vi "SOAE Main Panel.vi"(0 "Expt State (in)":T1) -> (4 "Expt State out":T1)   [LabVIEW 2020]
uses:
  Utility VIs/Type Defs/Left-Right ring.ctl
  CFTS Main Panel SubVIs/CFTS-Experiment State.ctl
  <vilib>/printing/EasyPrintingControls.llb/layout_options.ctl
  <vilib>/printing/EasyPrintingControls.llb/orientation.ctl
  <vilib>/printing/EasyPrintingControls.llb/panel_scaling_for_page.ctl
  <vilib>/printing/EasyPrintingControls.llb/margins.ctl
  <vilib>/printing/EasyPrintingControls.llb/margin_values.ctl
  <vilib>/printing/EasyPrintingControls.llb/measurement_system.ctl
  <vilib>/printing/EasyPrintingControls.llb/printer_options.ctl
  <vilib>/printing/EasyPrintingControls.llb/printing_method.ctl
  <vilib>/printing/EasyPrintingControls.llb/color_or_monochrome.ctl
  <vilib>/printing/EasyPrintingControls.llb/page_header_options.ctl
  <vilib>/printing/EasyPrintingControls.llb/page_headers.ctl
  <vilib>/printing/EasyPrintingControls.llb/page_header_content_options.ctl
  Utility VIs/Buttons/KCheckmarkBoolean 2.ctl
  Typedefs/SOAE-Options.ctl
  Typedefs/SOAE-Parameters.ctl
  Typedefs/SOAE-State.ctl
  <vilib>/printing/EasyPrintingControls.llb/contents.ctl
  <vilib>/printing/EasyPrinting.llb/Easy Print VI Panel or Documentation (refnum).vi
  <vilib>/Utility/NIReport.llb/NI_ReportGenerationCore.lvlib
panel:
  out "Acquired":i32
  in  "Save raw data":T2
  in  "layout options":T3={"orientation (unchanged)"=0, "panel scaling for page (unchanged)"=0, "margins"={"override VI margins (false)"=FALSE, "margins (1.00)"={"top"=1.0, "left"=1.0, "right"=1.0, "bottom"=1.0}, "measurement system (default)"=0}, "printer options"={"destination printer name (current)"="", "printing method (unchanged)"=0, "color or monochrome (unchanged)"=0}, "page header options"={"page headers (unchanged)"=0, "page header content options"={"Include VI Name"=TRUE, "Include VI Path"=TRUE, "Include Last Modification Date"=TRUE, "Include Date Printed"=TRUE, "Include Page Number"=TRUE, "Include VI Icon"=TRUE}}} {"page header options"."page headers (unchanged)" items=["Unchanged", "Include page headers", "Do not include page headers"]; "printer options"."color or monochrome (unchanged)" items=["Unchanged", "Color/grayscale", "Monochrome"]; "printer options"."printing method (unchanged)" items=["Unchanged", "Standard", "PostScript", "Bitmap"]; "panel scaling for page (unchanged)" items=["Unchanged", "No Scaling", "Scale front panel to fit"]; "orientation (unchanged)" items=["Unchanged", "portrait", "landscape"]; "margins"."measurement system (default)" items=["Default", "US", "Metric"]; "margins"."margins (1.00)"."right" format="%.2f"; "margins"."margins (1.00)"."bottom" format="%.2f"; "margins"."margins (1.00)"."top" format="%.2f"; "margins"."margins (1.00)"."left" format="%.2f"}
  in  "Params":T16={"Ear"=enum."Right", "Sampling rate (Hz)"=0.25, "Number of FFT points"=37, "Number of averages"=5.0, "Smoothing binwidth (Hz)"=300.0, "Mic gain (dB)"=5.0}
  in  "Start":bool
  in  "Stop":bool
  out "User":string
  out "Run #":string
  out "ID #":u16
  out "finished":errorcluster
  in  "Listbox":i32(listbox)
  out "Spectrum":cluster{"X":dbl[], "X":dbl[]}[](graph)
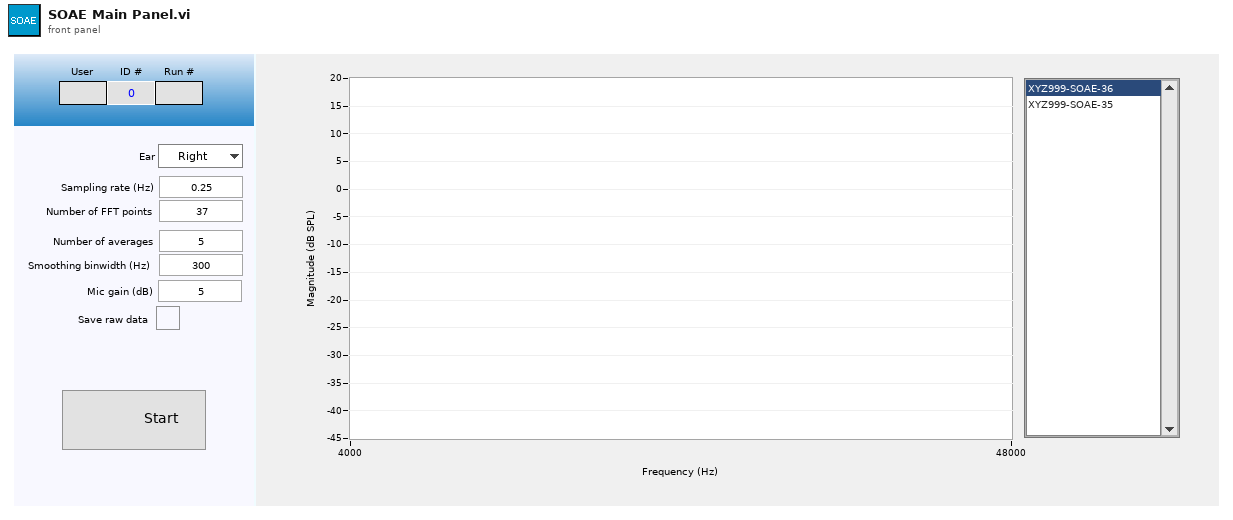
[diagram p1: front panel]
types:
  T1 = typedef "CFTS-Experiment State.ctl" = cluster{"Experimenter":string, "Number":u32, "Right":string, "Left":string, "Data Folder":path, "State File":path, "Version Info":string, "End Exposure Time":dbl, "Exposure Duration":string, "Run #":cluster{"CAP":i16, "ABR":i16, "DP":i16, "VsEP":i16, "MeasSeq":i16, "SubSeq":i16, "SFOAE":i16}}
  T2 = typedef "KCheckmarkBoolean 2.ctl" = bool
  T3 = typedef "NI_ReportGenerationCore.lvlib/layout_options.ctl" = cluster{"orientation (unchanged)":T4, "panel scaling for page (unchanged)":T5, "margins":T6, "printer options":T9, "page header options":T12}
  T4 = typedef "NI_ReportGenerationCore.lvlib/orientation.ctl" = u16
  T5 = typedef "NI_ReportGenerationCore.lvlib/panel_scaling_for_page.ctl" = u16
  T6 = typedef "NI_ReportGenerationCore.lvlib/margins.ctl" = cluster{"override VI margins (false)":bool, "margins (1.00)":T7, "measurement system (default)":T8}
  T7 = typedef "NI_ReportGenerationCore.lvlib/margin_values.ctl" = cluster{"top":dbl, "left":dbl, "right":dbl, "bottom":dbl}
  T8 = typedef "NI_ReportGenerationCore.lvlib/measurement_system.ctl" = u16
  T9 = typedef "NI_ReportGenerationCore.lvlib/printer_options.ctl" = cluster{"destination printer name (current)":string, "printing method (unchanged)":T10, "color or monochrome (unchanged)":T11}
  T10 = typedef "NI_ReportGenerationCore.lvlib/printing_method.ctl" = u16
  T11 = typedef "NI_ReportGenerationCore.lvlib/color_or_monochrome.ctl" = u16
  T12 = typedef "NI_ReportGenerationCore.lvlib/page_header_options.ctl" = cluster{"page headers (unchanged)":T13, "page header content options":T14}
  T13 = typedef "NI_ReportGenerationCore.lvlib/page_headers.ctl" = u16
  T14 = typedef "NI_ReportGenerationCore.lvlib/page_header_content_options.ctl" = cluster{"Include VI Name":bool, "Include VI Path":bool, "Include Last Modification Date":bool, "Include Date Printed":bool, "Include Page Number":bool, "Include VI Icon":bool}
  T15 = typedef "Left-Right ring.ctl" = enum16{"Right", "Left"}
  T16 = cluster{"Ear":T15, "Sampling rate (Hz)":dbl, "Number of FFT points":i32, "Number of averages":dbl, "Smoothing binwidth (Hz)":dbl, "Mic gain (dB)":dbl}
  T17 = typedef "SOAE-State.ctl" = cluster{"aborted":bool, "files":path[]}
  T18 = typedef "SOAE-Parameters.ctl" = cluster{"Ear":enum16{"Right", "Left"}, "Fs (Hz)":dbl, "Nfft":i32, "Navg":i32, "Binwidth (Hz)":dbl, "Gain (dB)":dbl}
  T19 = typedef "SOAE-Options.ctl" = cluster{"FreqScale":cluster{"Min":dbl, "Max":dbl}, "save raw":bool}
  T20 = typedef "SOAE-Acq Runtime.ctl" = cluster{"freq":dbl[], "raw":dbl[], "mag":dbl[], "pt":dbl[], "path":path, "task":refnum<k21>, "nacq":i32, "gain":dbl, "navg":i32, "stream":refnum<file>, "nread":i32, "fir":dbl[]}
  T21 = enum8{"Enabled", "Disabled", "Disabled and Grayed Out"}
  T22 = typedef "NI_ReportGenerationCore.lvlib/contents.ctl" = u16
  T23 = cluster{"Ear":T15, "Fs (Hz)":dbl, "Nfft":i32, "Number of averages":dbl, "Binwidth (Hz)":dbl, "Gain (dB)":dbl}
  T24 = cluster{"Params":cluster{"Ear":T15, "Fs (Hz)":dbl, "Nfft":i32, "Number of averages":dbl, "Binwidth (Hz)":dbl, "Gain (dB)":dbl}, "Path out":path, "save raw":bool}
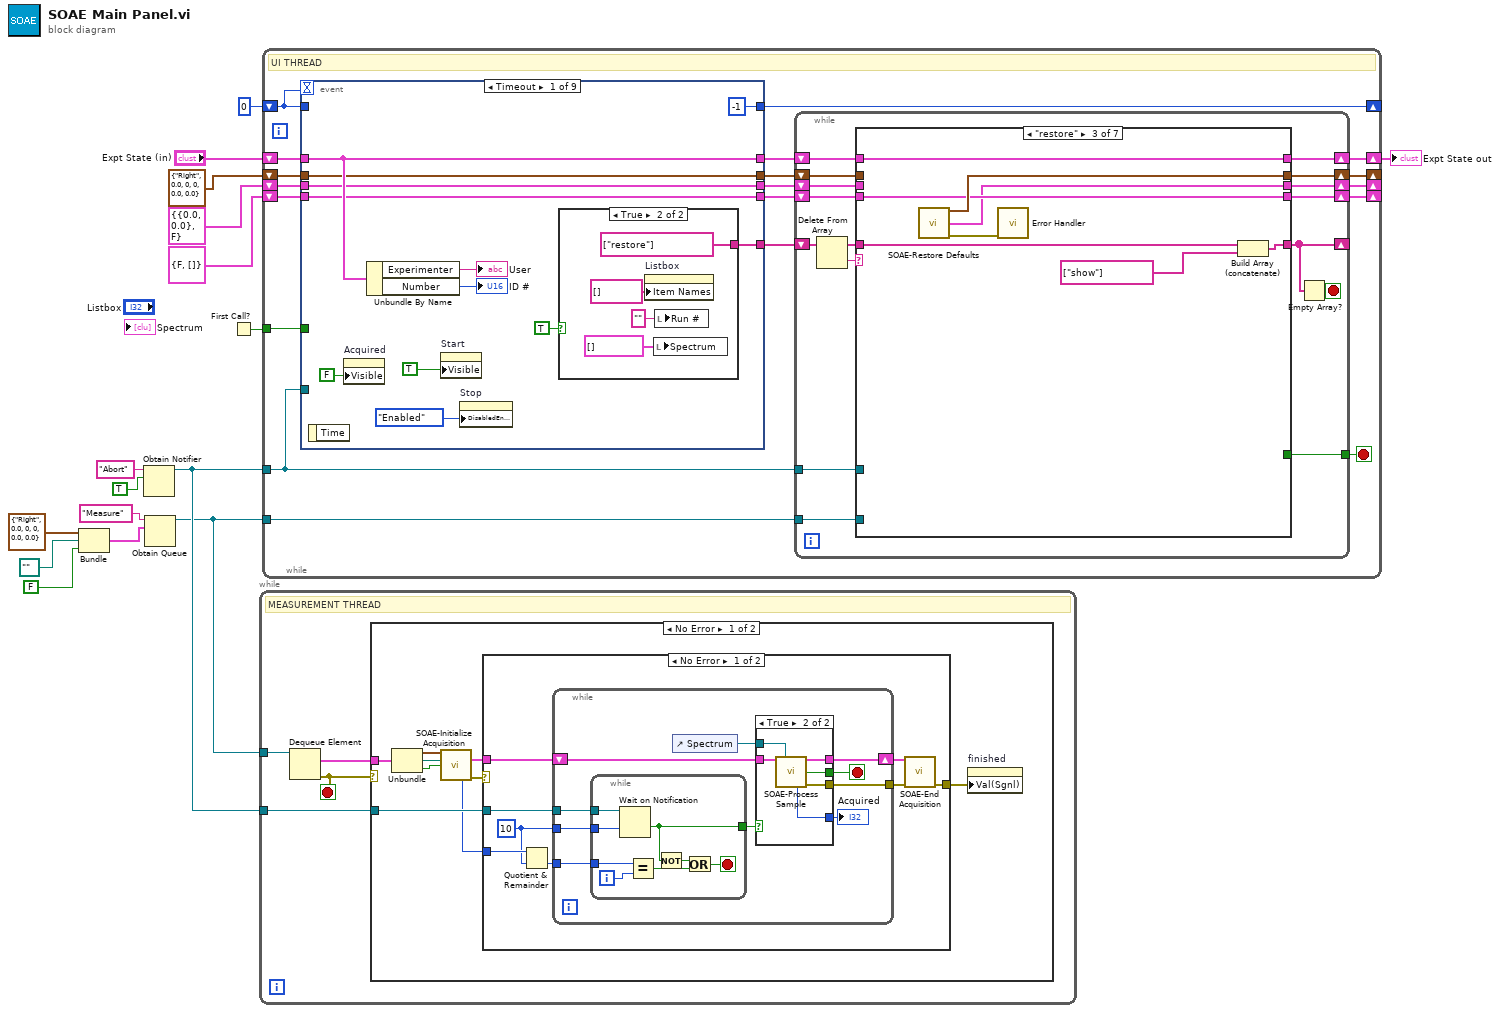
[diagram p0: block diagram]
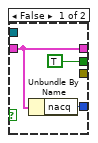
[diagram p2: hidden frame]
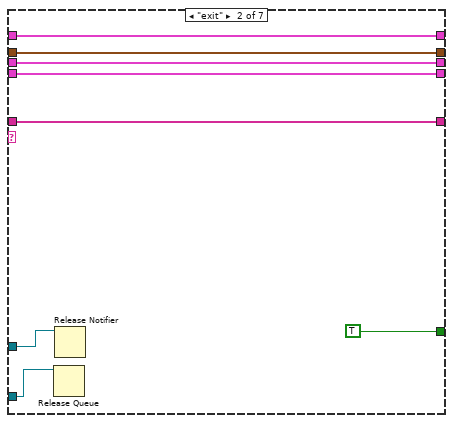
[diagram p6: hidden frame]
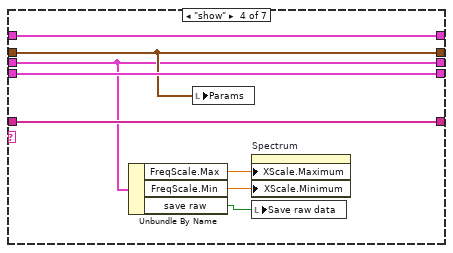
[diagram p7: hidden frame]
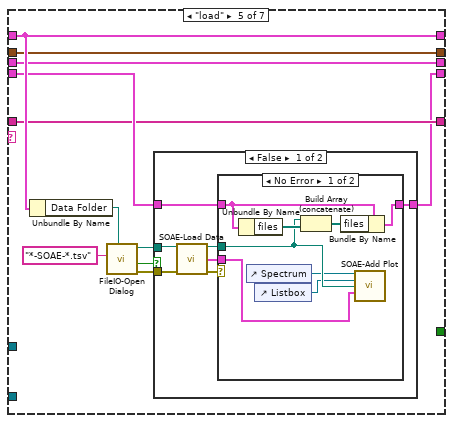
[diagram p8: hidden frame]
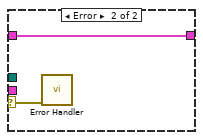
[diagram p9: hidden frame]
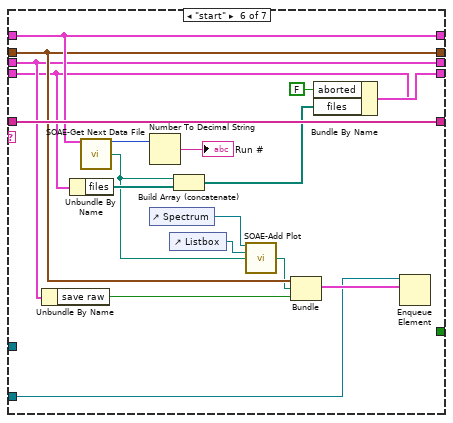
[diagram p11: hidden frame]
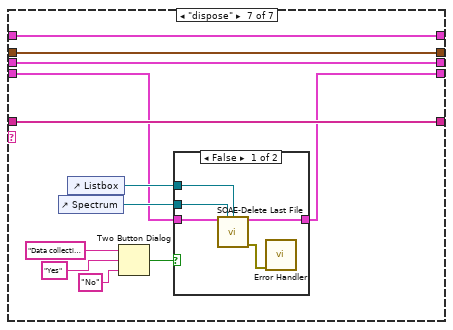
[diagram p12: hidden frame]
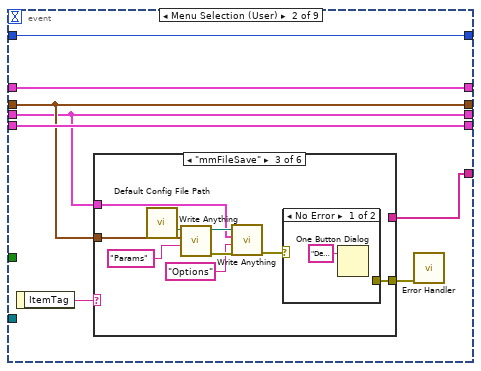
[diagram p15: hidden frame]
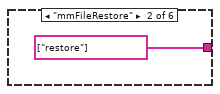
[diagram p17: hidden frame]
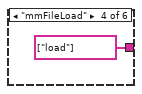
[diagram p19: hidden frame]
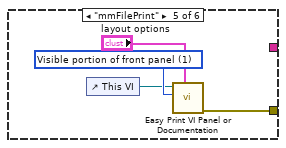
[diagram p20: hidden frame]
diagram:
  n1 = Bundle("Params"=T18 {"Ear"=enum."Right", "Fs (Hz)"=0.0, "Nfft"=0, "Navg"=0, "Binwidth (Hz)"=0.0, "Gain (dB)"=0.0}, path "", FALSE) -> (w12:cluster{"Params":T18, path, bool})  [unwired: 1 in]
  n2 = Obtain Notifier(name (unnamed)="Abort", notification data type=TRUE) -> (notifier out=w15:refnum<notifier>)  [unwired: 2 in, 2 out]
  n3 = Obtain Queue(name (unnamed)="Measure", element data type=w12) -> (queue out=w8:refnum<queue>)  [unwired: 3 in, 2 out]
  n4 = First Call?() -> (First Call?: T/F=w11:bool)
  n5 = while {
    tunnel: w8 -> [w20]
    tunnel: w15 -> [w17]
    stop <- w19 stop-if-true
    # "MEASUREMENT THREAD"
    n6 = Dequeue Element(queue=w20) -> (element=w18:cluster{"Params":T18, path, bool}, error out=w19:errorcluster)  [unwired: 2 in, 2 out]
    n7 = case shown="No Error" w19 {
      tunnel: w18 -> [w29 _]
      tunnel: w17 -> [w28 _]
      frame No Error {
        n8 = Unbundle(w29) -> ("Params"=w25:T18, w24:path, w27:bool)
        n9 = call "SOAE-Initialize Acquisition.vi"("Params"=w25, "Path"=w24, "raw data"=w27) -> ("runtime"=w23:T20, "T (ms)"=w22:u32, "error out"=w26:errorcluster)  [unwired: 10 in]
        n10 = case shown="No Error" w26 {
          selector: w26 -> [_ w65]
          tunnel: w28 -> [w37 _]
          tunnel: w23 -> [w36 _]
          tunnel: w22 -> [w35 _]
          tunnel: [w30 w65] -> w21
          frame No Error {
            w34 = 10 ("timeout in ms (-1)")
            n11 = Quotient & Remainder(x=w35, y=w34) -> (floor(x/y)=w33:u32)  [unwired: 1 out]
            n12 = while {
              shift-right: [w43] -> w31
              shift-left: w36 -> [w44]
              tunnel: w37 -> [w47]
              tunnel: w34 -> [w46]
              tunnel: w33 -> [w45]
              tunnel: [w40] -> w32
              stop <- w41 stop-if-true
              n13 = while {
                tunnel: [w58] -> w42
                tunnel: w46 -> [w63]
                tunnel: w45 -> [w62]
                tunnel: w47 -> [w64]
                i -> [w61]
                stop <- w59 stop-if-true
                n14 = Wait on Notification(notifier=w64, timeout in ms (-1)=w63) -> (timed out?=w58:bool)  [unwired: 2 in, 3 out]
                n15 = Equal?(x=w62, y=w61) -> (x = y?=w60:bool)
                n16 = Not(x=w58) -> (.not. x?=w57:bool)
                n17 = Or(x=w57, y=w60) -> (x .or. y?=w59:bool)
              }
              n18 = control-ref of="Spectrum"() -> (w39:refnum<vi>)
              n19 = case shown="True" w42 {
                tunnel: w44 -> [w49 w56]
                tunnel: [w49 w55] -> w43
                tunnel: [TRUE w53] -> w41
                tunnel: [_ w54] -> w40
                tunnel: w39 -> [_ w52]
                tunnel: [w48 w51] -> w38
                frame False {
                  n20 = Unbundle By Name(w49) -> ("nacq"=w48:i32)
                }
                frame True {
                  n21 = call "SOAE-Process Sample.vi"("runtime in"=w56, "Graph"=w52) -> ("runtime out"=w55:T20, "finished"=w53:bool, "acquired"=w51:i32, "error out"=w54:errorcluster)  [unwired: 10 in]
                }
              }
              "Acquired" <- w38
            }
            n22 = call "SOAE-End Acquisition.vi"("runtime"=w31, "error in (no error)"=w32) -> ("error out"=w30:errorcluster)  [unwired: 13 in]
          }
          frame Error {
          }
        }
        n23 = property on="finished" class="Clust (strict)"("Val(Sgnl)"=w21) -> ()  [unwired: 2 in, 2 out]
      }
      frame Error {
      }
    }
  }
  n24 = while {
    tunnel: w8 -> [w69]
    shift-right: [w84] -> _
    shift-left: 0 -> [w80]
    tunnel: w11 -> [w83]
    shift-right: [w75] -> w2
    shift-left: "Expt State (in)" -> [w82]
    shift-right: [w77] -> _
    shift-left: T18 {"Ear"=enum."Right", "Fs (Hz)"=0.0, "Nfft"=0, "Navg"=0, "Binwidth (Hz)"=0.0, "Gain (dB)"=0.0} ("Params") -> [w81]
    shift-right: [w71] -> _
    shift-left: T17 {"aborted"=FALSE, "files"=[]} ("State") -> [w73]
    tunnel: w15 -> [w70]
    shift-right: [w66] -> _
    shift-left: T19 {"FreqScale"={"Min"=0.0, "Max"=0.0}, "save raw"=FALSE} ("Options") -> [w68]
    stop <- w74 stop-if-true
    # "UI THREAD"
    n25 = event shown="[0] Timeout" {
      selector: _ -> [_ _ _ _ _ _ _ _ _]
      dyn-events: _ -> [_ _ _ _ _ _ _ _ _]
      timeout: w80 -> [_ _ w243 _ _ _ _ _ _]
      tunnel: [-1 w216 w243 w248 w255 w263 w274 w288 w297] -> w84
      tunnel: w83 -> [_ _ _ _ _ _ _ _ _]
      tunnel: w82 -> [w205 w215 w239 w247 w254 w262 w273 w287 w296]
      tunnel: [w205 w215 w239 w247 w254 w262 w273 w287 w296] -> w76
      tunnel: w81 -> [w204 w212 w241 _ w253 w264 w275 w286 w295]
      tunnel: [w204 w212 w241 "Params" w253 w264 w275 w286 w295] -> w78
      tunnel: w80 -> [_ w216 _ w248 w255 w263 w274 w288 w297]
      tunnel: [w200 w214 string[] ["exit"] ("f") _ _ string[] ["start"] ("f") _ w277 _] -> w79
      tunnel: w73 -> [w203 w213 w238 w246 w252 w260 w272 w281 w294]
      tunnel: [w203 w213 w238 w246 w252 w260 w267 w281 w294] -> w72
      tunnel: w70 -> [_ _ _ _ _ w259 w271 _ _]
      tunnel: w68 -> [w197 w211 w237 w244 w251 w258 w268 w285 w293]
      tunnel: [w197 w211 w237 w244 w250 w258 w268 w285 w292] -> w67
      event Timeout {
        n26 = event-data() -> ()  [unwired: 1 in, 1 out]
        n27 = property on="Acquired" class="DigNum (strict)"("Visible"=FALSE) -> ()  [unwired: 2 in, 2 out]
        n28 = Unbundle By Name(w205) -> ("Experimenter"=→"User":string, "Number"=→"ID #":u32)
        n29 = property on="Start" class="Bool"("Visible"=TRUE) -> ()  [unwired: 2 in, 2 out]
        n30 = property on="Stop" class="Bool"("DisabledEnum"=T21."Enabled" ("Disabled")) -> ()  [unwired: 2 in, 2 out]
        n31 = case shown="True" TRUE {
          tunnel: [_ string[] ["restore"]] -> w200
          frame False {
          }
          frame True {
            n32 = property on="Listbox" class="LstBox (strict)"("Item Names"=string[] []) -> ()  [unwired: 2 in, 2 out]
            n33 = local write "Spectrum"(cluster{"X":dbl[], "X":dbl[]}[] [] ("Spectrum")) -> ()
            n34 = local write "Run #"("" ("Run #")) -> ()
          }
        }
      }
      event Menu Selection (User) {
        n35 = event-data() -> ("ItemTag"=w218:string)  [unwired: 1 in]
        n36 = case shown="\"mmFileSave\"" w218 {
          tunnel: [_ _ w225 _ w232 _] -> w217
          tunnel: w212 -> [_ _ w226 _ _ _]
          tunnel: [_ string[] ["restore"] _ string[] ["load"] _ string[] ["exit"]] -> w214
          tunnel: w211 -> [_ _ w221 _ _ _]
          frame "", Default {
          }
          frame "mmFileRestore" {
          }
          frame "mmFileSave" {
            n37 = call "Default Config File Path.vi"() -> ("Default config file name"=w228:path)
            n38 = call "Write Anything.vi"("Section Name (Name of \"Anything\")"="Params" ("Section Name (Name of \"Anything\")"), "Anything"=w226, "Path (dialog)"=w228) -> ("Error Out"=w224:errorcluster, "Path out"=w223:path)  [unwired: 7 in]
            n39 = call "Write Anything.vi"("Error In"=w224, "Section Name (Name of \"Anything\")"="Options" ("Section Name (Name of \"Anything\")"), "Anything"=w221, "Path (dialog)"=w223) -> ("Error Out"=w220:errorcluster)  [unwired: 6 in, 1 out]
            n40 = case shown="No Error" w220 {
              selector: w220 -> [_ w230]
              tunnel: [_ w230] -> w225
              frame No Error {
                n41 = One Button Dialog(message="Defaults saved.") -> ()  [unwired: 1 in, 1 out]
              }
              frame Error {
              }
            }
          }
          frame "mmFileLoad" {
          }
          frame "mmFilePrint" {
            w234 = T22 1 items=["Complete front panel", "Visible portion of front panel", "Icon, description, panel and diagram", "Documentation: Using the panel", "Documentation: Using as a subVI", "Documentation: Complete", "Documentation: Custom"] ("contents (complete front panel)")
            n42 = control-ref of="This VI"() -> (w233:refnum<vi>)
            n43 = call-poly <vilib>:"Easy Print VI Panel or Documentation.vi"("layout options"="layout options", "contents (complete front panel)"=w234, "VI reference"=w233) -> ("error out"=w232:errorcluster)  [unwired: 7 in, 1 out]
          }
          frame "mmFileExit" {
          }
        }
        n44 = call "Error Handler.vi"("error in (no error)"=w217) -> ()  [unwired: 13 in, 2 out]
      }
      event Panel Close? {
        n45 = event-data() -> ()  [unwired: 1 in, 1 out]
        n46 = event-data("Discard?"=TRUE) -> ()  [unwired: 1 in, 1 out]
      }
      event "Params": Value Change {
        n47 = event-data() -> ()  [unwired: 1 in, 1 out]
      }
      event Value Change {
        n48 = event-data() -> ()  [unwired: 1 in, 1 out]
        n49 = Bundle By Name(cluster=w251, "save raw"="Save raw data") -> (w250:T19)
      }
      event "Start": Value Change {
        n50 = event-data() -> ()  [unwired: 1 in, 1 out]
        n51 = Cancel Notification(0:w259) -> ()  [unwired: 1 in, 3 out]
        n52 = property on="Start" class="Bool"("Visible"=FALSE) -> ()  [unwired: 2 in, 2 out]
        n53 = property on="Acquired" class="DigNum (strict)"("Visible"=TRUE) -> ()  [unwired: 2 in, 2 out]
        n54 = local write "Acquired"(0 ("Acquired")) -> ()
      }
      event "Stop": Value Change {
        n55 = event-data() -> ()  [unwired: 1 in, 1 out]
        n56 = Send Notification(notification=TRUE, notifier=w271) -> ()  [unwired: 1 in, 2 out]
        n57 = property on="Stop" class="Bool"("DisabledEnum"=T21."Disabled and Grayed Out" ("Disabled")) -> ()  [unwired: 2 in, 2 out]
        n58 = Bundle By Name(cluster=w272, "aborted"=TRUE) -> (w267:T17)
      }
      event "finished": Value Change {
        n59 = event-data() -> ("NewVal"=w279:errorcluster)  [unwired: 1 in]
        n60 = call "Error Handler.vi"("error in (no error)"=w279) -> ()  [unwired: 13 in, 2 out]
        n61 = property on="Start" class="Bool"("Visible"=TRUE) -> (error out=w284:errorcluster)  [unwired: 2 in, 1 out]
        n62 = Unbundle By Name(w281) -> ("aborted"=w280:bool)
        n63 = property on="Stop" class="Bool"(error in=w284, "DisabledEnum"=T21."Enabled" ("Disabled")) -> ()  [unwired: 1 in, 2 out]
        n64 = Or(x=w280, y=w279) -> (x .or. y?=w278:bool)
        n65 = case shown="True" w278 {
          tunnel: [_ string[] ["dispose"]] -> w277
          frame False {
          }
          frame True {
          }
        }
        n66 = property on="Acquired" class="DigNum (strict)"("Visible"=FALSE) -> ()  [unwired: 2 in, 2 out]
      }
      event "Spectrum": Scale Range Change {
        n67 = event-data() -> ("NewRange.Minimum"=w291:dbl, "NewRange.Maximum"=w290:dbl)  [unwired: 1 in]
        n68 = Bundle By Name(cluster=w293, "FreqScale.Min"=w291, "FreqScale.Max"=w290) -> (w292:T19)
      }
    }
    n69 = while {
      shift-right: [w90] -> _
      shift-left: w79 -> [w100]
      shift-right: [w93] -> w77
      shift-left: w78 -> [w96]
      shift-right: [w94] -> w75
      shift-left: w76 -> [w95]
      tunnel: w69 -> [w92]
      tunnel: [w91] -> w74
      shift-right: [w88] -> w71
      shift-left: w72 -> [w89]
      tunnel: w70 -> [w87]
      shift-right: [w85] -> w66
      shift-left: w67 -> [w86]
      stop <- w98 stop-if-true
      n70 = Delete From Array(array=w100) -> (deleted portion=w99:string, array with subset deleted=w97:string[])  [unwired: 2 in]
      n71 = case shown="\"restore\"" w99 {
        tunnel: w97 -> [w103 w112 w120 w128 w131 w176 w187]
        tunnel: w96 -> [w104 w113 _ w126 w133 w173 w188]
        tunnel: w95 -> [w105 w107 w121 w129 w139 w175 w185]
        tunnel: [w105 w107 w121 w129 w139 w175 w185] -> w94
        tunnel: [w104 w113 w118 w126 w133 w173 w188] -> w93
        tunnel: [w103 w112 w116 w128 w131 w176 w187] -> w90
        tunnel: w92 -> [_ w111 _ _ _ w169 _]
        tunnel: [_ TRUE _ _ _ _ _] -> w91
        tunnel: w89 -> [w102 w109 w117 w127 w135 w162 w178]
        tunnel: [w102 w109 w117 w127 w130 w164 w177] -> w88
        tunnel: w87 -> [_ w108 _ _ _ _ _]
        tunnel: w86 -> [w101 w106 _ w125 w132 w172 w186]
        tunnel: [w101 w106 w114 w125 w132 w172 w186] -> w85
        frame "", Default {
        }
        frame "exit" {
          n72 = Release Queue(queue=w111) -> ()  [unwired: 2 in, 3 out]
          n73 = Release Notifier(notifier=w108) -> ()  [unwired: 2 in, 3 out]
        }
        frame "restore" {
          n74 = call "SOAE-Restore Defaults.vi"() -> ("Params"=w118:T23, "Options"=w114:T19, "error out"=w119:errorcluster)  [unwired: 13 in]
          n75 = call "Error Handler.vi"("error in (no error)"=w119) -> ()  [unwired: 13 in, 2 out]
          n76 = Build Array (concatenate)(w120, string[] ["show"]) -> (w116:string[])
        }
        frame "show" {
          n77 = Unbundle By Name(w125) -> ("FreqScale.Max"=w124:dbl, "FreqScale.Min"=w123:dbl, "save raw"=w122:bool)
          n78 = local write "Params"(w126) -> ()
          n79 = property on="Spectrum" class="XYGraph (strict)"("XScale.Maximum"=w124, "XScale.Minimum"=w123) -> ()  [unwired: 2 in, 2 out]
          n80 = local write "Save raw data"(w122) -> ()
        }
        frame "load" {
          n81 = Unbundle By Name(w139) -> ("Data Folder"=w138:path)
          n82 = call "FileIO-Open Dialog.vi"("Default Folder"=w138, "pattern (all files)"="*-SOAE-*.tsv") -> ("error out"=w134:errorcluster, "cancelled"=w136:bool, "selected path"=w137:path)  [unwired: 7 in]
          n83 = case shown="False" w136 {
            tunnel: w137 -> [w146 _]
            tunnel: w135 -> [w147 w158]
            tunnel: w134 -> [w145 _]
            tunnel: [w141 w158] -> w130
            frame False {
              n84 = call "SOAE-Load Data.vi"("selected path"=w146, "error in (no error)"=w145) -> ("selected path out"=w142:path, "data"=w143:cluster{dbl[], dbl[]}, "error out"=w144:errorcluster)  [unwired: 10 in, 1 out]
              n85 = case shown="No Error" w144 {
                selector: w144 -> [_ w157]
                tunnel: w147 -> [w154 w156]
                tunnel: w143 -> [w148 _]
                tunnel: w142 -> [w151 _]
                tunnel: [w152 w156] -> w141
                frame No Error {
                  n86 = Unbundle By Name(w154) -> ("files"=w155:path[])
                  n87 = control-ref of="Spectrum"() -> (w150:refnum<vi>)
                  n88 = control-ref of="Listbox"() -> (w149:refnum<vi>)
                  n89 = Build Array (concatenate)(w151, w155) -> (w153:path[])
                  n90 = Bundle By Name(cluster=w154, "files"=w153) -> (w152:T17)
                  n91 = call "SOAE-Add Plot.vi"("Graph"=w150, "Listbox"=w149, "Path in"=w151, "XY Data"=w148) -> ()  [unwired: 11 in, 1 out]
                }
                frame Error {
                  n92 = call "Error Handler.vi"("error in (no error)"=w157) -> ()  [unwired: 13 in, 2 out]
                }
              }
            }
            frame True {
            }
          }
        }
        frame "start" {
          n93 = Unbundle By Name(w172) -> ("save raw"=w171:bool)
          n94 = Unbundle By Name(w162) -> ("files"=w160:path[])
          n95 = call "SOAE-Get Next Data File.vi"("Expt State"=w175) -> ("Run #"=w174:i32, "Path"=w159:path)  [unwired: 13 in]
          n96 = Number To Decimal String(number=w174) -> (decimal integer string=→"Run #":string)  [unwired: 1 in]
          n97 = control-ref of="Spectrum"() -> (w168:refnum<vi>)
          n98 = control-ref of="Listbox"() -> (w167:refnum<vi>)
          n99 = Build Array (concatenate)(w159, w160) -> (w161:path[])
          n100 = call "SOAE-Add Plot.vi"("Graph"=w168, "Listbox"=w167, "Path in"=w159) -> ("Path out"=w166:path)  [unwired: 12 in]
          n101 = Bundle("Params"=w173, "Path out"=w166, "save raw"=w171) -> (w170:T24)  [unwired: 1 in]
          n102 = Bundle By Name(cluster=w162, "aborted"=FALSE, "files"=w161) -> (w164:T17)
          n103 = Enqueue Element(queue=w169, element=w170) -> ()  [unwired: 2 in, 3 out]
        }
        frame "dispose" {
          n104 = control-ref of="Spectrum"() -> (w180:refnum<vi>)
          n105 = control-ref of="Listbox"() -> (w179:refnum<vi>)
          n106 = Two Button Dialog(message="Data collection aborted. Save data?", 1:"No" ("F button name (\"Cancel\")"), 2:"Yes" ("T button name (\"OK\")")) -> (T button?=w181:bool)
          n107 = case shown="False" w181 {
            tunnel: w180 -> [w191 _]
            tunnel: w178 -> [w193 w194]
            tunnel: w179 -> [w192 _]
            tunnel: [w190 w194] -> w177
            frame False {
              n108 = call "SOAE-Delete Last File.vi"("State"=w193, "XYGraph in"=w191, "Listbox"=w192) -> ("State out"=w190:T17, "error out"=w189:errorcluster)  [unwired: 11 in]
              n109 = call "Error Handler.vi"("error in (no error)"=w189) -> ()  [unwired: 13 in, 2 out]
            }
            frame True {
            }
          }
        }
      }
      n110 = Empty Array?(array=w90) -> (empty?=w98:bool)
    }
  }
  "Expt State out" <- w2
